vi "Fake nav.vi"(7 "Overall speed":dbl, 8 "stop":bool, 9 "Make start deg 0":bool, 10 "Array":dbl[][](array[numeric]), 11 "FPGA VI Reference In":T1) -> ()   [LabVIEW 2012]
uses:
  Compass/Compass IO.lvlib
  <vilib>/Analysis/NI_AAL_Angle.lvlib
  <vilib>/Analysis/coordinate.llb/Angle Range (Degree).ctl
  Globals.vi
  <vilib>/Analysis/coordinate.llb/Angle Units.ctl
  FPGA_ref.ctl
panel:
  in  "Start up":u32=20000
  out "No more Waypoints":bool
  out "Ang vol":sgl
  out "Y speed":dbl
  out "X speed":dbl
  in  "Waypoint":i16
  # "Ignore Front ir"
  # "Heading"
  # "Forward Speed"
  # "Time (ms)"
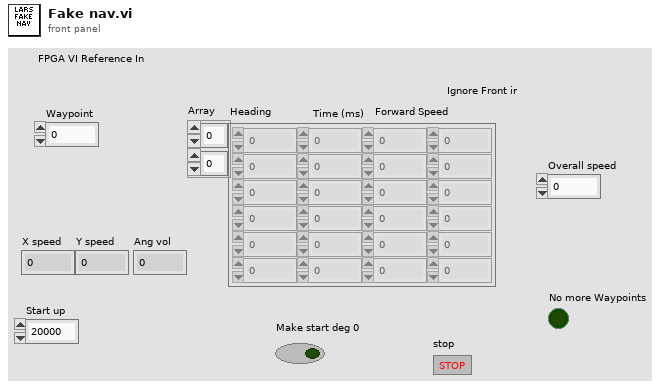
[diagram p1: front panel]
types:
  T1 = typedef "FPGA_ref.ctl" = refnum<k20>
  T2 = typedef "NI_AAL_Angle.lvlib/Angle Units.ctl" = i32
  T3 = typedef "NI_AAL_Angle.lvlib/Angle Range (Degree).ctl" = u16
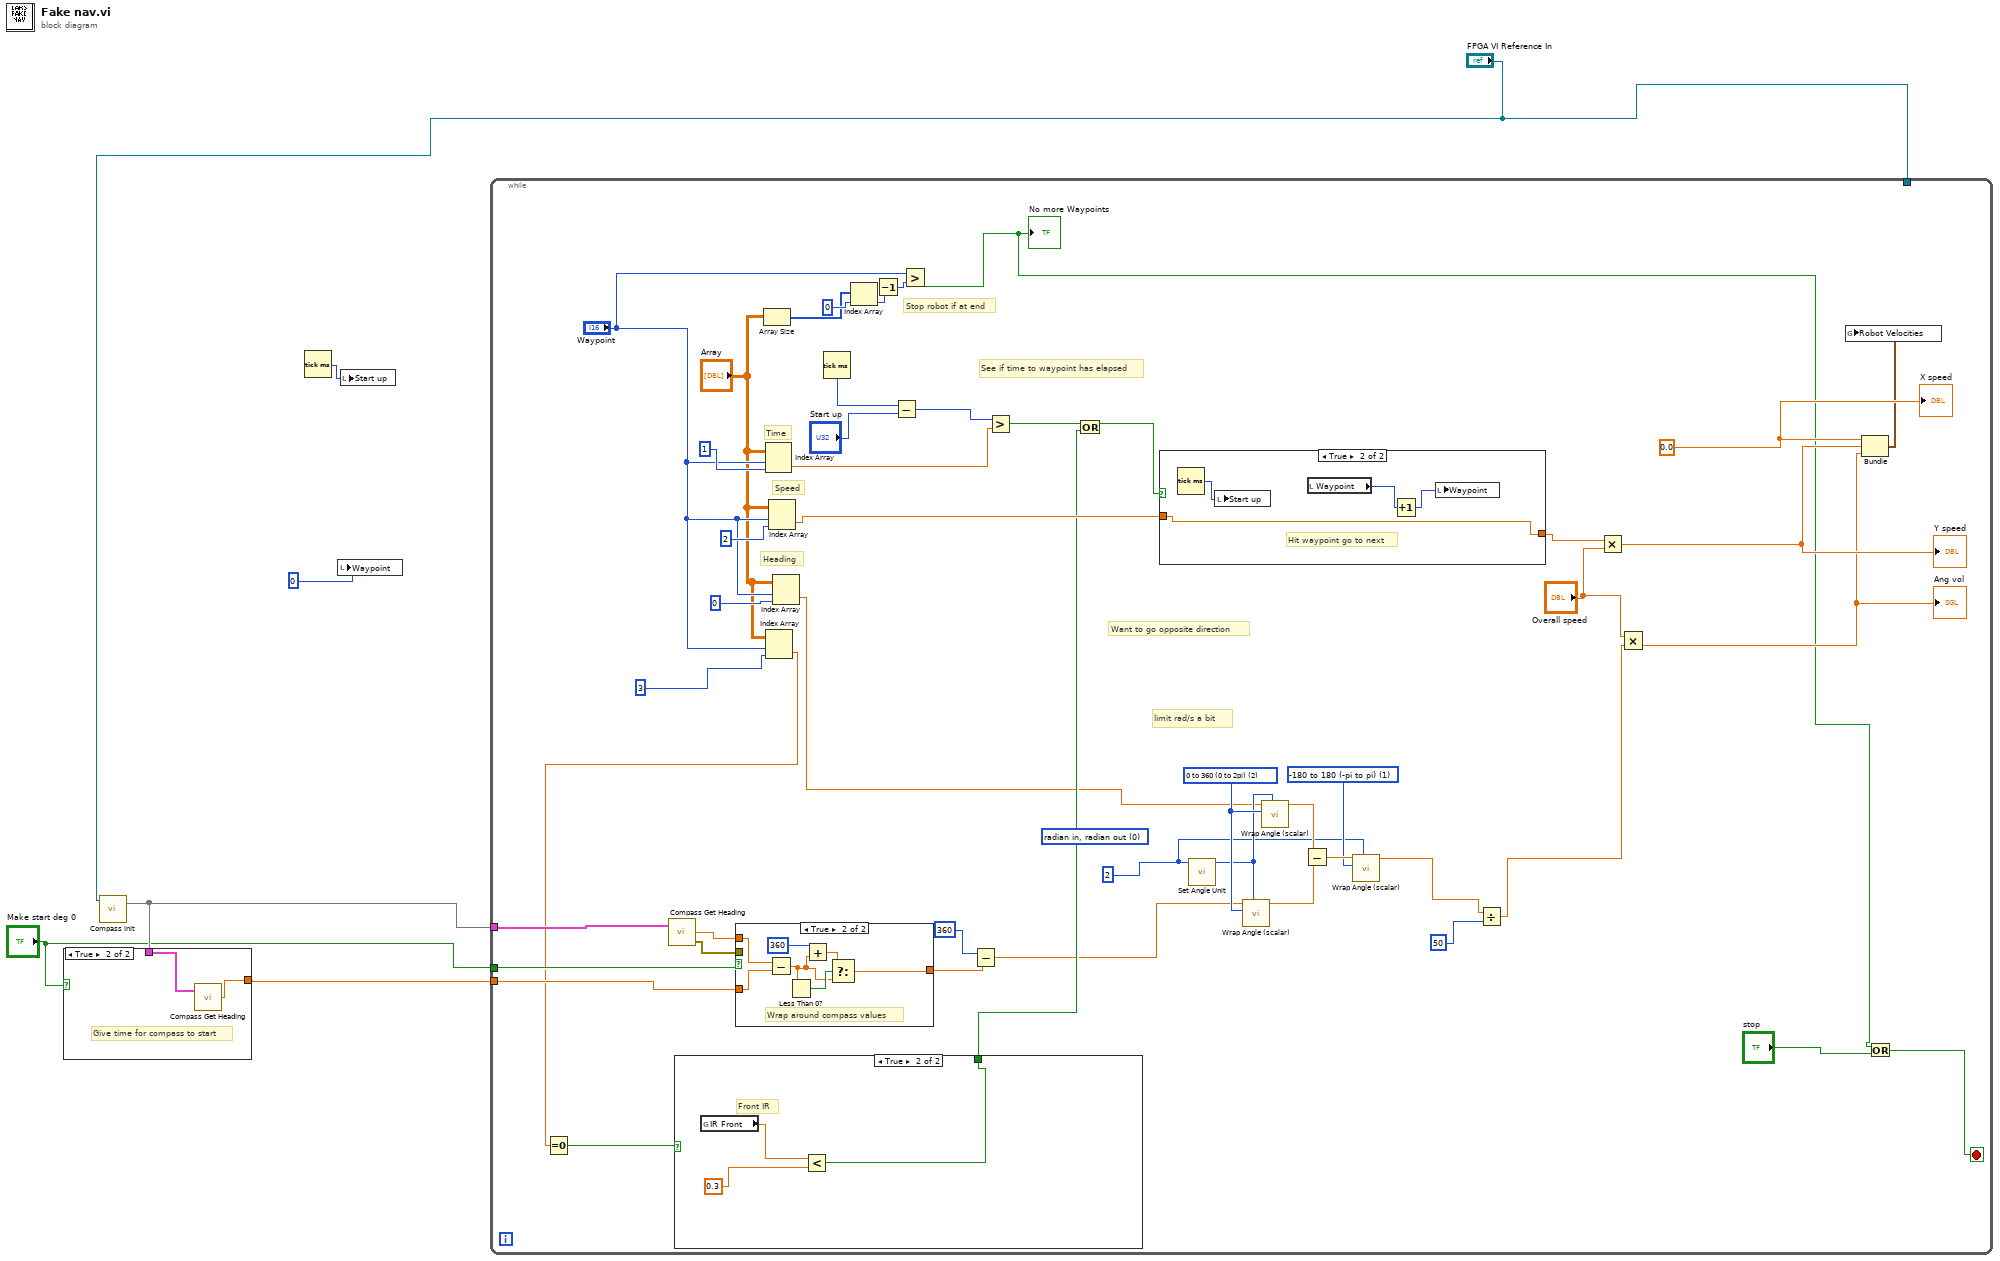
[diagram p0: block diagram]
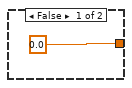
[diagram p2: hidden frame]
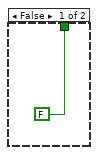
[diagram p3: hidden frame]
diagram:
  n1 = call "Compass Init.vi"("FPGA VI Reference"="FPGA VI Reference In") -> (1:w6)  [unwired: 3 in, 1 out]
  n2 = case shown="True" "Make start deg 0" {
    tunnel: w6 -> [_ w9]
    tunnel: [sgl 0.0 w8] -> w4
    frame False {
    }
    frame True {
      # "Give time for compass to start"
      n3 = call "Compass Get Heading.vi"("FPGA Information In"=w9) -> ("Heading (deg)"=w8:dbl)  [unwired: 2 in, 1 out]
    }
  }
  n4 = Tick Count (ms)() -> (millisecond timer value=w1:u32)
  n5 = local write "Waypoint"(0) -> ()
  n6 = local write "Start up"(w1) -> ()
  n7 = while {
    tunnel: w6 -> [w42]
    tunnel: "Make start deg 0" -> [w41]
    tunnel: w4 -> [w40]
    tunnel: "FPGA VI Reference In" -> [_]
    stop <- w38 stop-if-true
    (unwired) T2 0 items=["radian in, radian out", "radian in, degree out", "degree in, degree out", "degree in, radian out"] ("angle units in")
    w23 = 2
    w25 = T3 1 items=["none", "-180 to 180 (-pi to pi)", "0 to 360 (0 to 2pi)"] ("angle range")
    w29 = T3 2 items=["none", "-180 to 180 (-pi to pi)", "0 to 360 (0 to 2pi)"] ("angle range")
    w46 = 0.0
    # "Speed"
    # "limit rad/s a bit"
    # "Want to go opposite direction"
    # "Time"
    # "Heading"
    # "See if time to waypoint has elapsed"
    # "Stop robot if at end"
    n8 = call "Compass Get Heading.vi"("FPGA Information In"=w42) -> ("Heading (deg)"=w35:dbl, "error out"=w31:errorcluster)  [unwired: 2 in]
    n9 = case shown="True" w41 {
      tunnel: w35 -> [w62 w69]
      tunnel: w40 -> [_ w68]
      tunnel: [w62 w63] -> w34
      tunnel: w31 -> [_ _]
      frame False {
      }
      frame True {
        # "Wrap around compass values"
        n10 = Subtract(x=w69, y=w68) -> (x-y=w66:dbl)
        n11 = Less Than 0?(x=w66) -> (x < 0?=w67:bool)
        n12 = Add(x=u32 360, y=w66) -> (x+y=w65:dbl)
        n13 = Select(t=w65, s=w67, f=w66) -> (s? t:f=w63:dbl)
      }
    }
    n14 = Array Size(array="Array") -> (size(s)=w52:i32[])
    n15 = Index Array(array="Array", index (row)="Waypoint", index (col)=1) -> (element=w50:dbl)
    n16 = Index Array(array="Array", index (row)="Waypoint", index (col)=3 ("index (row)")) -> (element=w14:dbl)
    n17 = Equal To 0?(x=w14) -> (x = 0?=w15:bool)
    n18 = case shown="True" w15 {
      tunnel: [FALSE w60] -> w12
      frame False {
      }
      frame True {
        # "Front IR"
        n19 = global read "Globals.vi" "IR Front"() -> (w59:dbl)
        n20 = Less?(x=w59, y=0.3) -> (x < y?=w60:bool)
      }
    }
    n21 = Index Array(array="Array", index (row)="Waypoint", index (col)=2) -> (element=w47:dbl)
    n22 = Index Array(array="Array", index (row)="Waypoint", index (col)=0) -> (element=w11:dbl)
    n23 = Tick Count (ms)() -> (millisecond timer value=w36:u32)
    n24 = Index Array(array=w52, index=0) -> (element=w54:i32)
    n25 = Decrement(x=w54) -> (x-1=w51:i32)
    n26 = Subtract(x=w36, y="Start up") -> (x-y=w30:u32)
    n27 = Greater?(x="Waypoint", y=w51) -> (0:w39:bool)
    "No more Waypoints" <- w39
    n28 = Subtract(x=u32 360, y=w34) -> (x-y=w10:dbl)
    n29 = Greater?(x=w30, y=w50) -> (0:w49:bool)
    n30 = Or(x=w49, y=w12) -> (x .or. y?=w13:bool)
    n31 = case shown="True" w13 {
      tunnel: [w70 w72] -> w57
      tunnel: w47 -> [w70 w72]
      frame False {
      }
      frame True {
        # "Hit waypoint go to next"
        n32 = Tick Count (ms)() -> (millisecond timer value=w71:u32)
        n33 = local write "Start up"(w71) -> ()
        n34 = local read "Waypoint"() -> (w74:i16)
        n35 = Increment(x=w74) -> (x+1=w73:i16)
        n36 = local write "Waypoint"(w73) -> ()
      }
    }
    n37 = call <vilib>:"Set Angle Unit.vi"("angle units in"=w23) -> ("angle units out"=w24:T2)  [unwired: 10 in]
    n38 = call <vilib>:"Wrap Angle (scalar).vi"("angle units"=w24, "angle range"=w29, "angle in"=w10) -> ("angle out"=w27:dbl)  [unwired: 7 in, 1 out]
    n39 = call <vilib>:"Wrap Angle (scalar).vi"("angle units"=w24, "angle range"=w29, "angle in"=w11) -> ("angle out"=w28:dbl)  [unwired: 7 in, 1 out]
    n40 = Subtract(x=w28, y=w27) -> (x-y=w26:dbl)
    n41 = call <vilib>:"Wrap Angle (scalar).vi"("angle units"=w23, "angle range"=w25, "angle in"=w26) -> ("angle out"=w22:dbl)  [unwired: 7 in, 1 out]
    n42 = Divide(x=w22, y=50) -> (x/y=w21:dbl)
    n43 = Multiply(x=w57, y="Overall speed") -> (x*y=w45:dbl)
    "Y speed" <- w45
    n44 = Multiply(x="Overall speed", y=w21) -> (x*y=w44:dbl)
    "Ang vol" <- w44
    n45 = Bundle(w46, w45, w44) -> (w19:cluster{dbl, dbl, dbl})  [unwired: 1 in]
    n46 = global write "Globals.vi" "Robot Velocities"(w19) -> ()
    n47 = Or(x=w39, y="stop") -> (x .or. y?=w38:bool)
    "X speed" <- w46
  }
